vi "Image2WallDistances.vi"(3 "error in (no error)":errorcluster, 5 "Image Src":T3) -> (0 "error out":errorcluster, 2 "Walls":T1(array[cluster]))   [LabVIEW 2009, in "ImageAnalysis.lvlib"]
uses:
  ImageAnalysis.lvlib
  <vilib>/vision/Image Controls.llb/IMAQ Image.ctl
  <vilib>/vision/Shape Detection.llb/ShapeDetectionMatchOptions.ctl
  <vilib>/vision/Pattern Matching.llb/IMAQ Match Range Setting.ctl
  ImageProcessing.lvlib
  <vilib>/vision/NI_Vision_Development_Module.lvlib
  ControlProject/NetworkVarTarget.lvlib
panel:
  in  "Wall":T2
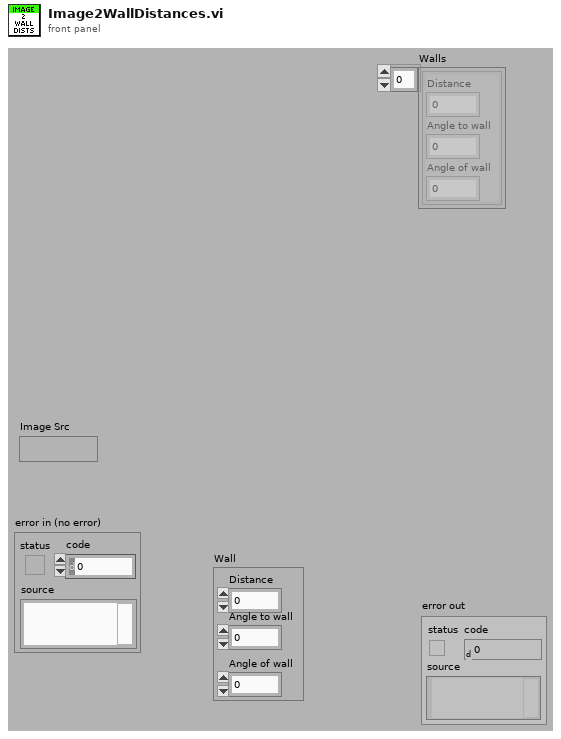
[diagram p1: front panel]
types:
  T1 = cluster{"Distance":dbl, "Angle to wall":dbl, "Angle of wall":dbl}[]
  T2 = cluster{"Distance":dbl, "Angle to wall":dbl, "Angle of wall":dbl}
  T3 = typedef "IMAQ Image.ctl" = refnum<image>
  T4 = typedef "ShapeDetectionMatchOptions.ctl" = cluster{"Rotation":bool, "Scale":bool, "Occlusion":bool, "Range Settings":T5[]}
  T5 = typedef "IMAQ Match Range Setting.ctl" = cluster{"Match Constraints":u32, "Min":dbl, "Max":dbl}
  T6 = cluster{"Min Major Radius":dbl, "Max Major Radius":dbl, "Min Minor Radius":dbl, "Max Minor Radius":dbl}
  T7 = cluster{"Position":cluster{"X":sgl, "Y":sgl}, "Angle":dbl, "Major Radius":dbl, "Minor Radius":dbl, "Score":dbl}[]
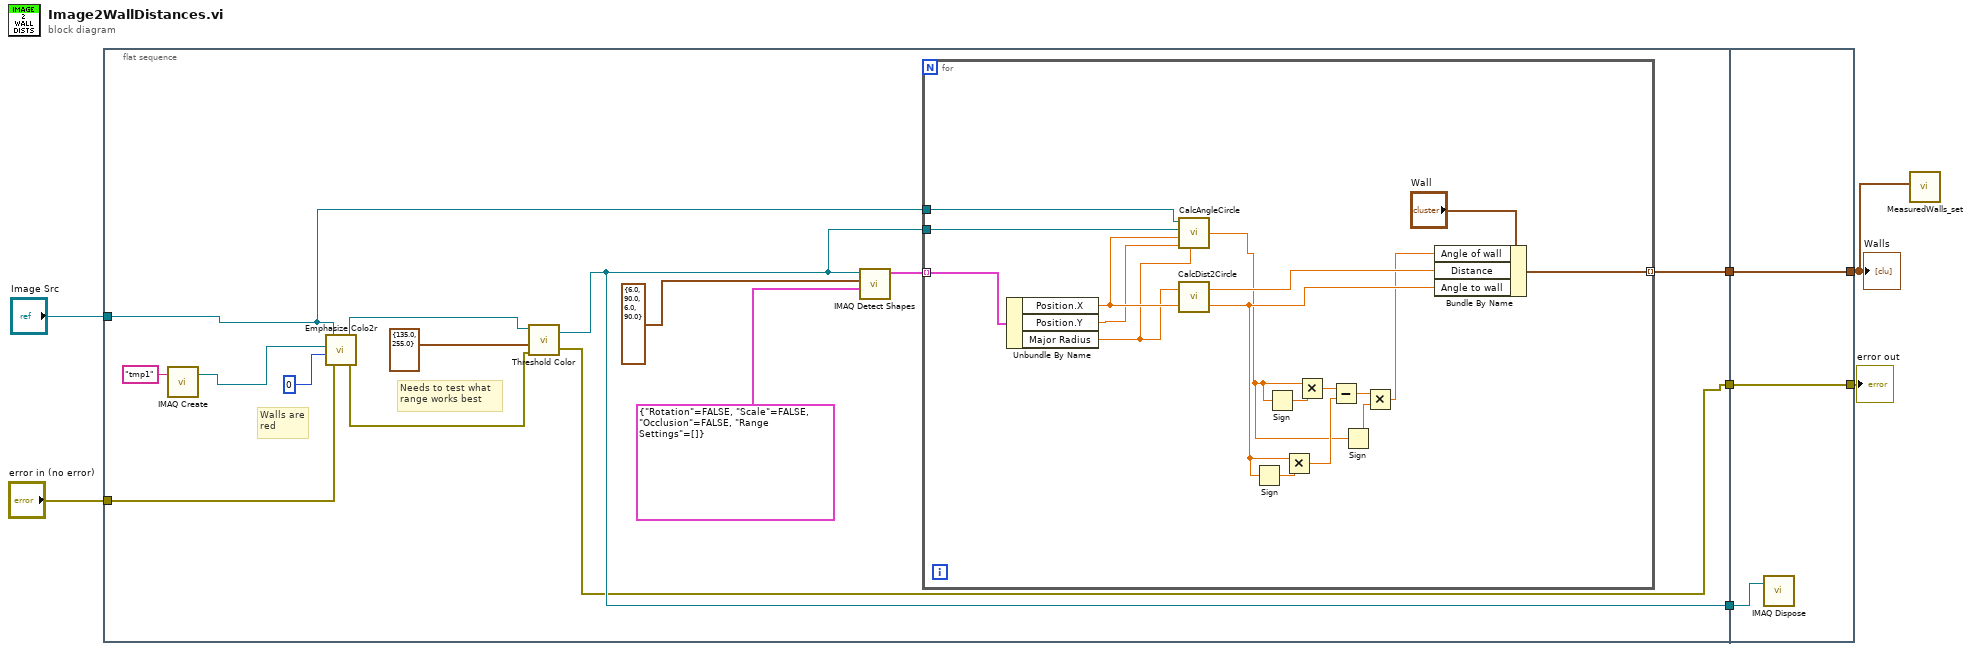
[diagram p0: block diagram]
diagram:
  n1 = flat-sequence {
    tunnel: "Image Src" -> [w14]
    tunnel: "error in (no error)" -> [w16]
    tunnel: [w10] -> w5
    tunnel: [w13] -> w3
    tunnel: [w11] -> w2
    tunnel: w5 -> [w42]
    tunnel: [w42] -> w4
    tunnel: [w41] -> w1
    tunnel: w3 -> [w41]
    tunnel: w2 -> [w40]
    frame #0 {
      # "Needs to test what \nrange works best"
      # "Walls are\nred"
      n2 = call "IMAQ Create"("Image Name"="tmp1") -> ("New Image"=w17:T3)  [unwired: 4 in, 1 out]
      n3 = call "Emphasize Colo2r.vi"("error in (no error)"=w16, "Color"=i8 0, "Image Dst"=w17, "Image Src"=w14) -> ("error out"=w21:errorcluster, "Image Out"=w12:T3)
      n4 = call "Threshold Color.vi"("error in (no error)"=w21, "Range"=cluster{"Lower value":sgl, "Upper value":sgl} {"Lower value"=135.0, "Upper value"=255.0}, "Image Src"=w12) -> ("error out"=w10:errorcluster, "Image Dst Out"=w11:T3)  [unwired: 1 in]
      n5 = call-poly "IMAQ Detect Shapes"("Match Options"=T4 {"Rotation"=FALSE, "Scale"=FALSE, "Occlusion"=FALSE, "Range Settings"=[]}, "Ellipse Descriptor"=T6 {"Min Major Radius"=6.0, "Max Major Radius"=90.0, "Min Minor Radius"=6.0, "Max Minor Radius"=90.0}, "Image"=w11) -> ("Ellipses"=w15:T7)  [unwired: 6 in, 2 out]
      n6 = for {
        tunnel: w15 -> [w39] mode=indexing
        tunnel: w11 -> [w38]
        tunnel: w14 -> [w34]
        tunnel: [w31] -> w13 mode=indexing
        n7 = Unbundle By Name(w39) -> ("Position.X"=w37:sgl, "Position.Y"=w36:sgl, "Major Radius"=w35:dbl)
        n8 = call "CalcAngleCircle.vi"("Original Image"=w34, "Filtered Image"=w38, "X Coordinate"=w37, "Y Coordinate"=w36, "Vertical radius"=w35) -> ("Angle in rad"=w23:dbl)
        n9 = call "CalcDist2Circle.vi"("X-cords"=w37, "Height of circle"=w35) -> ("Angle to circle"=w28:dbl, "Distance"=w32:dbl)
        n10 = Sign(1:w28) -> (0:w29:dbl)
        n11 = Sign(1:w23) -> (0:w30:dbl)
        n12 = Multiply(x=w28, y=w29) -> (x*y=w26:dbl)
        n13 = Multiply(x=w23, y=w30) -> (x*y=w27:dbl)
        n14 = Subtract(x=w27, y=w26) -> (x-y=w25:dbl)
        n15 = Sign(1:w23) -> (0:w24:dbl)
        n16 = Multiply(x=w25, y=w24) -> (x*y=w22:dbl)
        n17 = Bundle By Name(cluster="Wall", "Angle of wall"=w22, "Distance"=w32, "Angle to wall"=w28) -> (w31:T2)
      }
    }
    frame #1 {
      n18 = call "IMAQ Dispose"("Image"=w40) -> ()  [unwired: 5 in, 1 out]
    }
  }
  n19 = call "MeasuredWalls_set.vi"("MeasuredWalls"=w1) -> ()  [unwired: 10 in, 1 out]
  "error out" <- w4
  "Walls" <- w1
